vi "Add Remove Test.vi"() -> (0 "error out":errorcluster, 2 "Success Delete":bool, 3 "Success ADD":bool)   [LabVIEW 2015, in "SystemLink File Module tests.lvlib"]
doc: "Tests the Add Line and Remove Line functions."
uses:
  SystemLink File Module tests.lvlib
  <vilib>/NI/Tag Bus/tag/Data Type.ctl
  module/configuration/Line.ctl
  <vilib>/NI/Tag Bus Module Framework/channel/TBM channel.lvclass
  module/configuration/Data Tag Type.ctl
  module/configuration/permissions.ctl
  module/configuration/SystemLink File configuration.lvclass
  <vilib>/NI/Tag Bus/tag/tag descriptor.lvclass
panel:
  out "Deleted Line":string
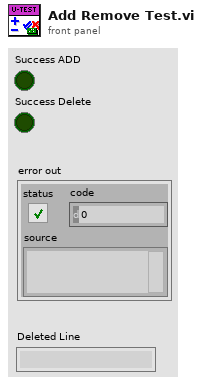
[diagram p1: front panel]
types:
  T1 = typedef "SystemLink File configuration.lvclass/permissions.ctl" = enum32{"Read from SystemLink", "Write to SystemLink"}
  T2 = typedef "SystemLink File configuration.lvclass/Line.ctl" = cluster{"channel":refnum<class "TBM channel.lvclass">, "Data Tag Type":T3}
  T3 = typedef "SystemLink File configuration.lvclass/Data Tag Type.ctl" = enum16{"Double", "Single", "I32", "I16", "I8", "U64", "U32", "U16", "U8", "Boolean", "String", "Timestamp"}
  T4 = typedef "tag bus.lvlib/tag descriptor.lvclass/Data Type.ctl" = enum16{"Double", "Single", "I64", "I32", "I16", "I8", "U64", "U32", "U16", "U8", "Boolean", "String", "Array of Double", "Array of Single", "Array of I64", "Array of I32", "Array of I16", "Array of I8", "Array of U64", "Array of U32", "Array of U16", "Array of U8", "Array of Boolean", "Array of String"}
  T5 = typedef "TBM channel.lvclass/channel classification.ctl" = enum16{"input data", "output data", "processing parameter", "processing result"}
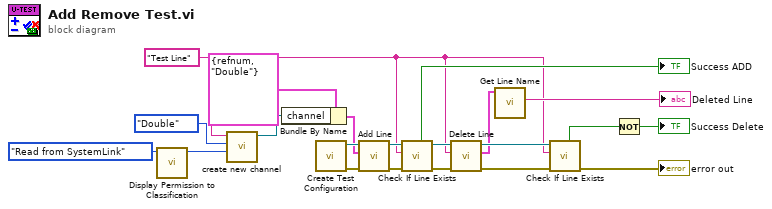
[diagram p0: block diagram]
diagram:
  w1 = "Test Line" ("channel name")
  n1 = call "Display Permission to Classification.vi"("display permissions"=permissions."Read from SystemLink") -> ("channel classification"=w19:T5)  [unwired: 10 in]
  n2 = call <vilib>:"create new channel.vi"("channel classification"=w19, "data type"=Data_Type."Double", "channel name"=w1) -> ("channel"=w20:refnum<class "TBM channel.lvclass">)  [unwired: 8 in]
  n3 = Bundle By Name(cluster=T2 {"channel"=refnum, "Data Tag Type"=enum."Double"} ("Line"), "channel"=w20) -> (w17:T2)
  n4 = call "Create Test Configuration.vi"() -> ("error out"=w10:errorcluster, "Module Configuration"=w21:refnum<class "SystemLink File configuration.lvclass">)  [unwired: 6 in, 4 out]
  n5 = call "Add Line.vi"("error in"=w10, "Line"=w17, "SystemLin Tag Module configuration in"=w21) -> ("error out"=w12:errorcluster, "SystemLin Tag Module configuration out"=w15:refnum<class "SystemLink File configuration.lvclass">)  [unwired: 6 in, 1 out]
  n6 = call-dynamic "Check If Line Exists.vi"("error in"=w12, "Name to Locate"=w1, "SystemLin Tag Module configuration in"=w15) -> ("error out"=w11:errorcluster, "SystemLin Tag Module configuration out"=w14:refnum<class "SystemLink File configuration.lvclass">, "Found?"=→"Success ADD":bool)  [unwired: 4 in, 2 out]
  n7 = call "Delete Line.vi"("error in"=w11, "Line Name"=w1, "SystemLin Tag Module configuration in"=w14) -> ("error out"=w9:errorcluster, "Deleted Line"=w3:T2, "SystemLin Tag Module configuration out"=w7:refnum<class "SystemLink File configuration.lvclass">)  [unwired: 6 in]
  n8 = call "Get Line Name.vi"("Line in"=w3) -> ("Name"=→"Deleted Line":string)  [unwired: 8 in, 2 out]
  n9 = call-dynamic "Check If Line Exists.vi"("error in"=w9, "Name to Locate"=w1, "SystemLin Tag Module configuration in"=w7) -> ("error out"=→"error out":errorcluster, "Found?"=w6:bool)  [unwired: 4 in, 3 out]
  n10 = Not(x=w6) -> (.not. x?=→"Success Delete":bool)
